vi "Init Camera.vi"() -> (2 "Video Q out":refnum<queue>, 3 "Camera out":T1)   [LabVIEW 2012]
uses:
  <vilib>/userdefined/High Color/IMAQdx.ctl
  <vilib>/vision/driver/NI_Vision_Acquisition_Software.lvlib
  <resource>/objmgr/imaqdx.rc
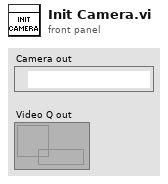
[diagram p1: front panel]
types:
  T1 = typedef "IMAQdx.ctl" = refnum<k21>
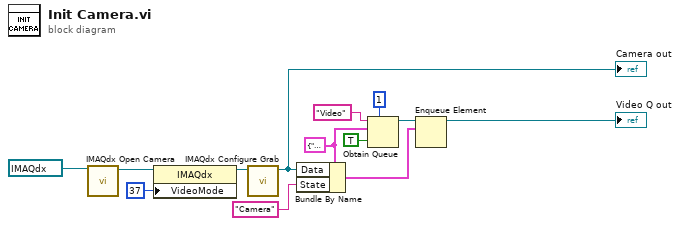
[diagram p0: block diagram]
diagram:
  w7 = cluster{"State":string, "Data":variant} {"State"="", "Data"=variant} ("State Cluster")
  n1 = call <vilib>:"IMAQdx Open Camera.vi"("Session In"=T1 "cam1") -> ("Session Out"=w11:T1)  [unwired: 9 in, 1 out]
  n2 = property class="IMAQdx"(reference=w11, "VideoMode"=u32 37) -> (reference out=w12:T1)  [unwired: 1 in, 1 out]
  n3 = call <vilib>:"IMAQdx Configure Grab.vi"("Session In"=w12) -> ("Session Out"=w9:T1)  [unwired: 9 in, 1 out]
  "Camera out" <- w9
  n4 = Bundle By Name(cluster=w7, "Data"=w9, "State"="Camera") -> (w6:cluster{"State":string, "Data":variant})
  n5 = Obtain Queue(max queue size (-1, unlimited)=1, name (unnamed)="Video", element data type=w7, create if not found? (T)=TRUE) -> (queue out=w5:refnum<queue>)  [unwired: 1 in, 2 out]
  n6 = Enqueue Element(queue=w5, element=w6) -> (queue out=→"Video Q out":refnum<queue>)  [unwired: 2 in, 2 out]
